vi "SUB_TestSound_Format.vi"(4 "Receiving Ai Name":string, 5 "Sending Ao Name":string, 6 "SPEC THD %":dbl, 7 "SPEC Max Sound Level":dbl, 8 "SPEC Min Sound Level":dbl, 9 "SPEC TXRX Diff HZ":dbl, 10 "Test Freq(HZ)":string, 11 "Test Item":string) -> (3 "output cluster":T1)   [LabVIEW 2011]
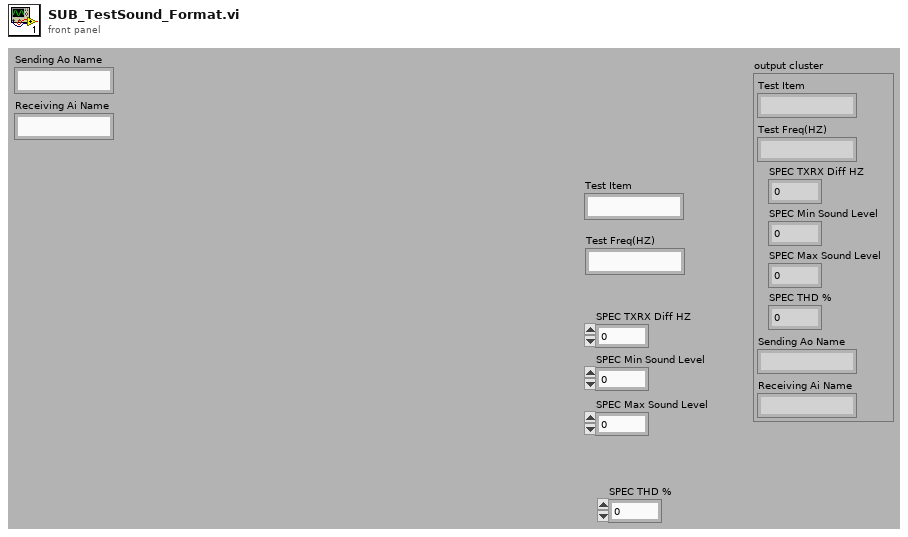
[diagram p1: front panel]
types:
  T1 = cluster{"Test Item":string, "Test Freq(HZ)":string, "SPEC TXRX Diff HZ":dbl, "SPEC Min Sound Level":dbl, "SPEC Max Sound Level":dbl, "SPEC THD %":dbl, "Sending Ao Name":string, "Receiving Ai Name":string}
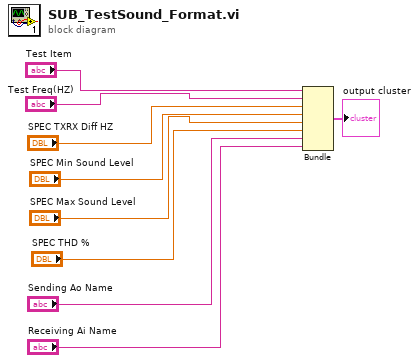
[diagram p0: block diagram]
diagram:
  n1 = Bundle("Test Item"="Test Item", "Test Freq(HZ)"="Test Freq(HZ)", "SPEC TXRX Diff HZ"="SPEC TXRX Diff HZ", "SPEC Min Sound Level"="SPEC Min Sound Level", "SPEC Max Sound Level"="SPEC Max Sound Level", "SPEC THD %"="SPEC THD %", "Sending Ao Name"="Sending Ao Name", "Receiving Ai Name"="Receiving Ai Name") -> (→"output cluster":T1)  [unwired: 1 in]
